vi "GPS_XY_Convert.vi"(8 "error in (no error)":errorcluster caption="错误输入（无错误）", 9 "纬度":string, 11 "经度":string) -> (0 "转换之后的纬度2":string, 1 "转换之后的经度2":string, 2 "转换后的纬度":string, 3 "转换后的经度":string, 4 "error out":errorcluster caption="错误输出")   [LabVIEW 2018]
uses:
  <vilib>/httpClient/LabVIEWHTTPClient.lvlib
panel:
  out "子字符串之后":string
  out "body":string caption="体部"
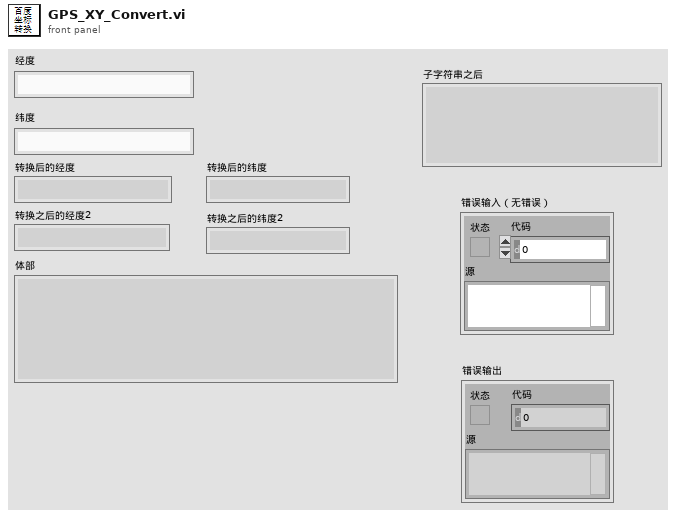
[diagram p1: front panel]
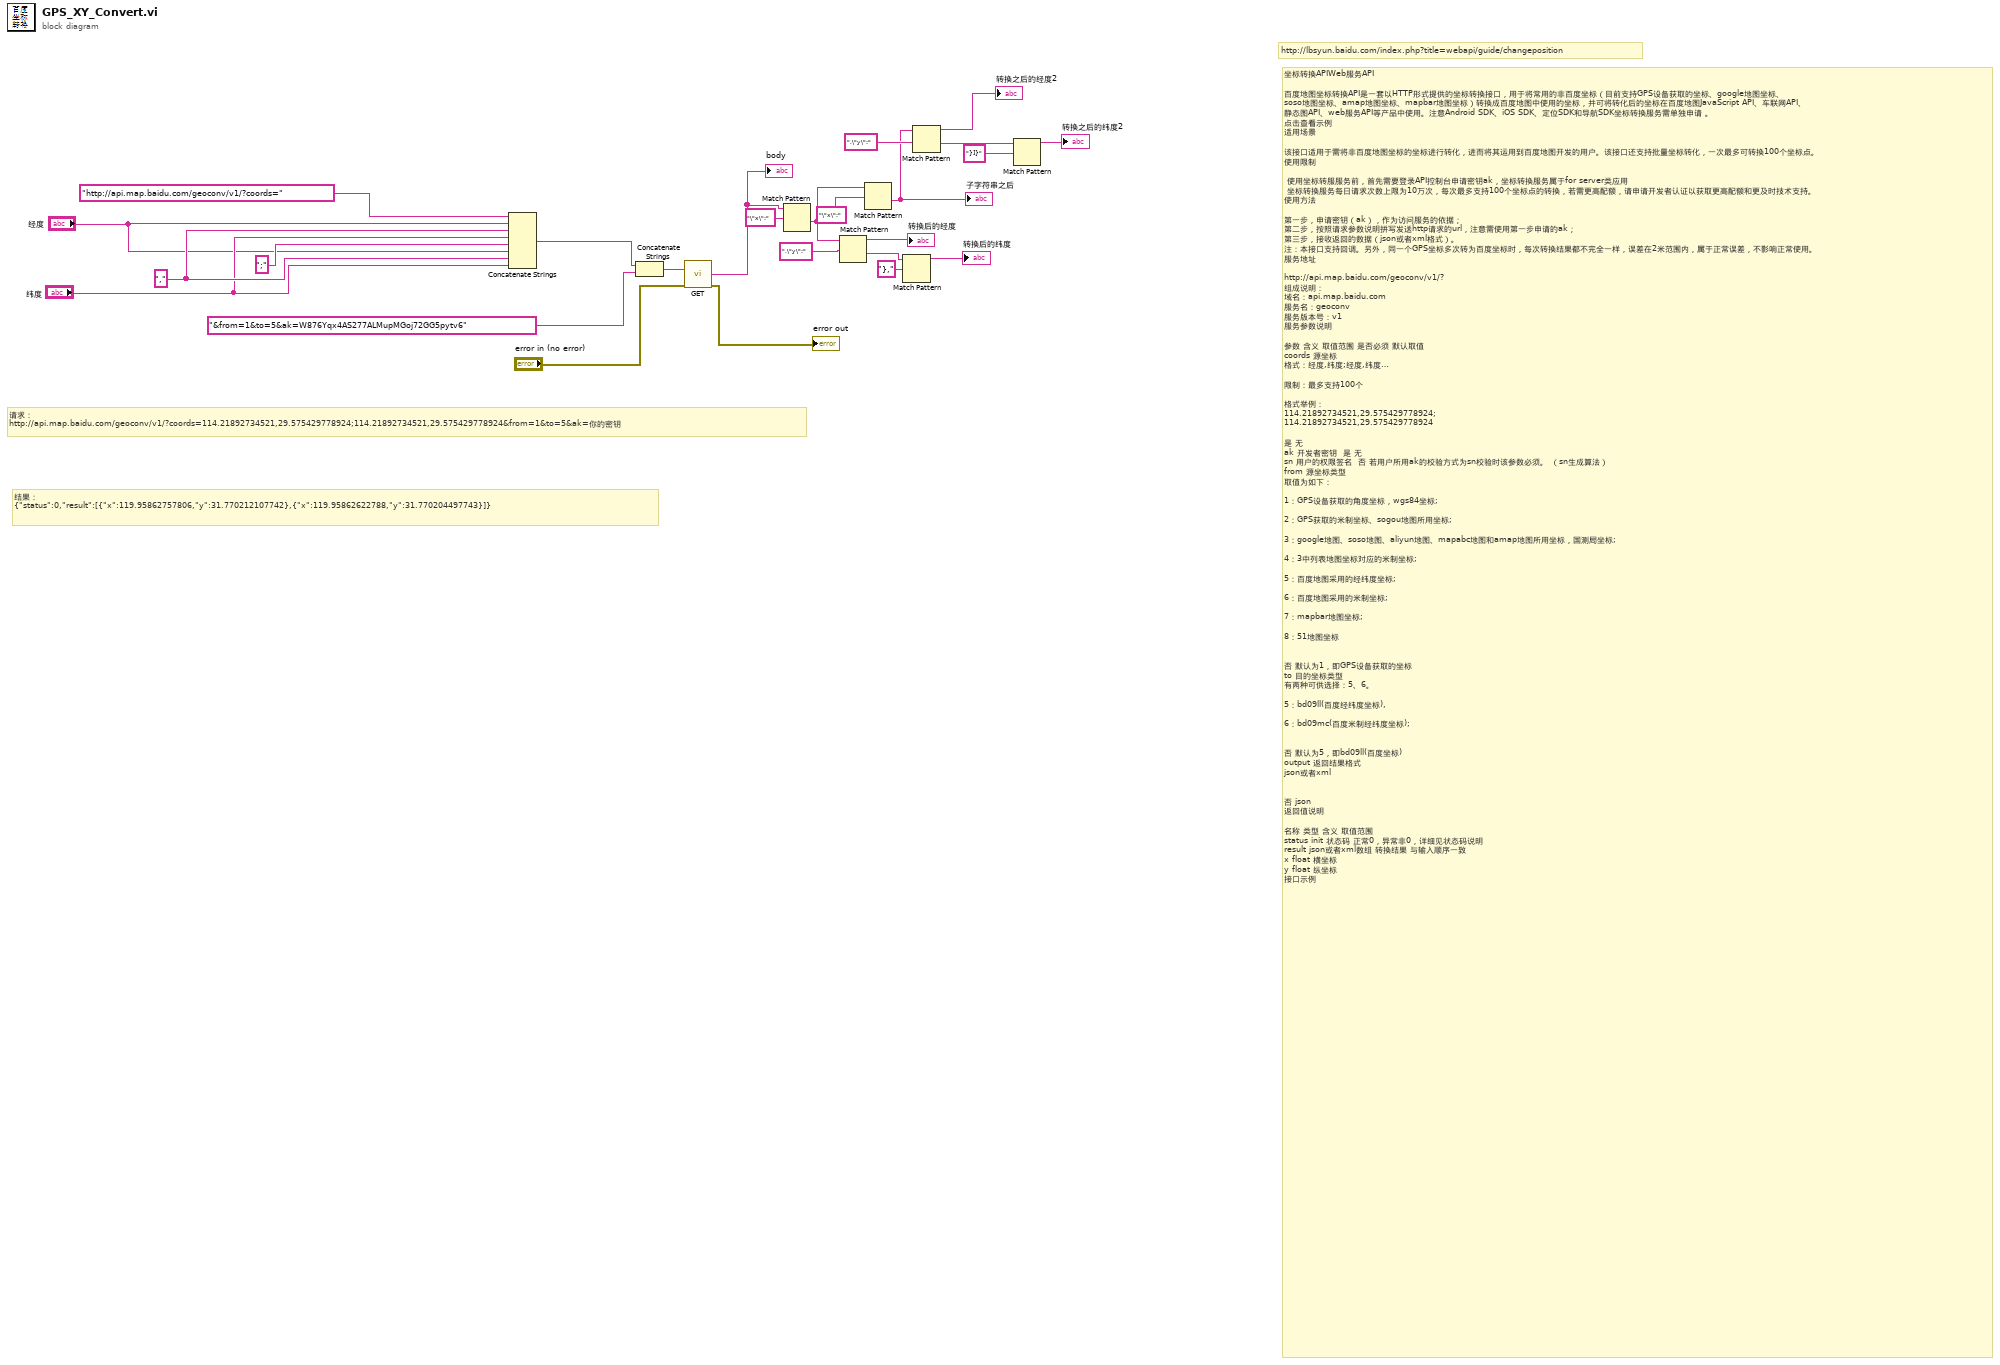
[diagram p0: block diagram]
diagram:
  w23 = ","
  # "结果：\n{\"status\":0,\"result\":[{\"x\":119.95862757806,\"y\":31.770212107742},{\"x\":119.95862622788,\"y\":31.770204497743}]}"
  # "请求：\nhttp://api.map.baidu.com/geoconv/v1/?coords=114.21892734521,29.575429778924;114.21892734521,29.575429778924&from=1&to=5&ak=你的密钥"
  # "坐标转换APIWeb服务API\n\n百度地图坐标转换API是一套以HTTP形式提供的坐标转换接口，用于将常用的非百度坐标（目前支持GPS设备获取的坐标、google地图坐标、\nsoso地图坐标、amap地图坐标、mapbar地图坐标）转换成百度地图中使用的坐标，并可将转化后的坐标在百度地图JavaScript API、车联网API、\n静态图API、web服务API等产品中使用。注意Android SDK、iOS SDK、定位SDK和导航SDK坐标转换服务需单独申请 。\n点击查看示例\n适用场景\n\n该接口适用于需将非百度地图坐标的坐标进行转化，进而将其运用到百度地图开发的用户。该接口还支持批量坐标转化，一次最多可转换100个坐标点。\n使用限制\n\n 使用坐标转服服务前，首先需要登录API控制台申请密钥ak，坐标转换服务属于for server类应用\n 坐标转换服务每日请求次数上限为10万次，每次最多支持100个坐标点的转换，若需更高配额，请申请开发者认证以获取更高配额和更及时技术支持。\n使用方法\n\n第一步，申请密钥（ak），作为访问服务的依据；\n第二步，按照请求参数说明拼写发送http请求的url，注意需使用第一步申请的ak；\n第三步，接收返回的数据（json或者xml格式）。\n注：本接口支持回调。另外，同一个GPS坐标多次转为百度坐标时，每次转换结果都不完全一样，误差在2米范围内，属于正常误差，不影响正常使用。\n服务地址\n\nhttp://api.map.baidu.com/geoconv/v1/?\n组成说明：\n域名：api.map.baidu.com\n服务名：geoconv\n服务版本号：v1\n服务参数说明\n\n参数\t含义\t取值范围\t是否必须\t默认取值\ncoords\t源坐标\t\n格式：经度,纬度;经度,纬度…\n\n限制：最多支持100个\n\n格式举例：\n114.21892734521,29.575429778924;\n114.21892734521,29.575429778924\n\n是\t无\nak\t开发者密钥\t\t是\t无\nsn\t用户的权限签名\t\t否\t若用户所用ak的校验方式为sn校验时该参数必须。 （sn生成算法）\nfrom\t源坐标类型\t\n取值为如下：\n\n1：GPS设备获取的角度坐标，wgs84坐标;\n\n2：GPS获取的米制坐标、sogou地图所用坐标;\n\n3：google地图、soso地图、aliyun地图、mapabc地图和amap地图所用坐标，国测局坐标;\n\n4：3中列表地图坐标对应的米制坐标;\n\n5：百度地图采用的经纬度坐标;\n\n6：百度地图采用的米制坐标;\n\n7：mapbar地图坐标;\n\n8：51地图坐标\n\n\n否\t默认为1，即GPS设备获取的坐标\nto\t目的坐标类型\t\n有两种可供选择：5、6。\n\n5：bd09ll(百度经纬度坐标),\n\n6：bd09mc(百度米制经纬度坐标);\n\n\n否\t默认为5，即bd09ll(百度坐标)\noutput\t返回结果格式\t\njson或者xml\n\n\n否\tjson\n返回值说明\n\n名称\t类型\t含义\t取值范围\nstatus\tinit\t状态码\t正常0，异常非0，详细见状态码说明\nresult\tjson或者xml数组\t转换结果\t与输入顺序一致\nx\tfloat\t横坐标\t\ny\tfloat\t纵坐标\t\n接口示例"
  # "http://lbsyun.baidu.com/index.php?title=webapi/guide/changeposition"
  n1 = Concatenate Strings("http://api.map.baidu.com/geoconv/v1/?coords=" ("字符串"), "经度", w23, "纬度", ";" ("字符串"), "经度", w23, "纬度") -> (w22:string)
  n2 = Concatenate Strings(w22, "&from=1&to=5&ak=W876Yqx4AS277ALMupMGoj72GG5pytv6" ("字符串")) -> (w20:string)
  n3 = call <vilib>:"GET.vi"("url"=w20, "error in (no error)"="error in (no error)") -> ("body"=w19:string, "error out"=→"error out":errorcluster)  [unwired: 10 in, 2 out]
  "body" <- w19
  n4 = Match Pattern(string=w19, regular expression="\"x\":" ("正则表达式")) -> (after substring=w8:string)  [unwired: 1 in, 3 out]
  n5 = Match Pattern(string=w8, regular expression=",\"y\":" ("正则表达式")) -> (before substring=→"转换后的经度":string, after substring=w11:string)  [unwired: 1 in, 2 out]
  n6 = Match Pattern(string=w8, regular expression="\"x\":" ("正则表达式")) -> (after substring=w5:string)  [unwired: 1 in, 3 out]
  "子字符串之后" <- w5
  n7 = Match Pattern(string=w11, regular expression="}," ("正则表达式")) -> (before substring=→"转换后的纬度":string)  [unwired: 1 in, 3 out]
  n8 = Match Pattern(string=w5, regular expression=",\"y\":" ("正则表达式")) -> (before substring=→"转换之后的经度2":string, after substring=w2:string)  [unwired: 1 in, 2 out]
  n9 = Match Pattern(string=w2, regular expression="}]}" ("正则表达式")) -> (before substring=→"转换之后的纬度2":string)  [unwired: 1 in, 3 out]
